vi "Export Configuation.vi"() -> ()   [LabVIEW 2015, in "J1939 Addon System Explorer.lvlib"]
uses:
  J1939 Addon System Explorer.lvlib
  <vilib>/NI Veristand/Custom Device API/Custom Device Item Ref.ctl
  <vilib>/NI/NIVS System Definition Utilities/System Definition Utilities.lvlib
  <vilib>/NI VeriStand/Custom Device API/Custom Device API.lvlib
panel:
  out "error out":errorcluster
  in  "Node Ptr":T1=18446744073709551615 format="%.0x"
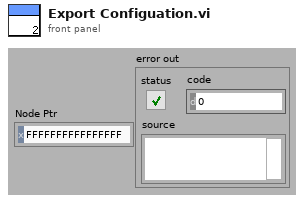
[diagram p1: front panel]
types:
  T1 = typedef "Custom Device API.lvlib/Custom Device Item Ref.ctl" = u64
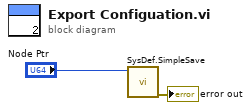
[diagram p0: block diagram]
diagram:
  n1 = call <vilib>:"SysDef.SimpleSave.vi"("ID"="Node Ptr") -> ("error out"=→"error out":errorcluster)  [unwired: 9 in, 1 out]
